vi "RW_main.vi"(0 "Rotating Wall Parameters":T1={"Start Frequency"=20000.0, "Stop Frequency"=20000.0, "Sweep Time"=0.0, "Amplitude"=1.5, "Phase (ch.1)"=0.001, "Phase (Ch.2)"=90.0} {"Sweep Time" format="%.4f"; "Phase (Ch.2)" min=-1800.0 max=1800.0 step=0.1 format="%.3f"; "Phase (ch.1)" min=-1800.0 max=1800.0 step=0.1 format="%.3f"; "Stop Frequency" format="%#.5p"; "Start Frequency" format="%#.5p"; "Amplitude" min=0.0 max=4.0 format="%.3f"}, 1 "On/Off":bool, 2 "VISAsession":refnum<visa-resource-name>="wavefactoryU10") -> ()   [LabVIEW 2018]
panel:
  out "x-y 5":u32=300
  out "x-y 4":u32=100
  out "x-y 3":u32=901
  out "x-y 2":u32=800
  out "x-y":u32=600
  out "millisecond timer value":u32=88672931
  out "error out":errorcluster caption="Error OUT"
  # "Turn-on\nTimes (ms)"
  # "Turn-off\nTimes (ms)"
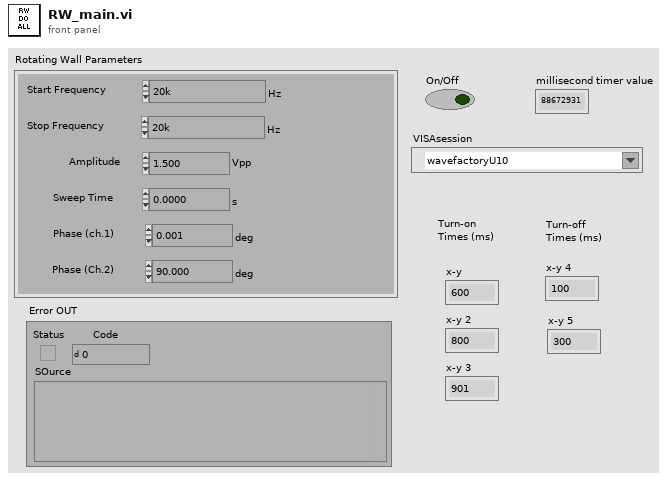
[diagram p1: front panel]
types:
  T1 = cluster{"Start Frequency":dbl, "Stop Frequency":dbl, "Sweep Time":dbl, "Amplitude":dbl, "Phase (ch.1)":dbl, "Phase (Ch.2)":dbl}
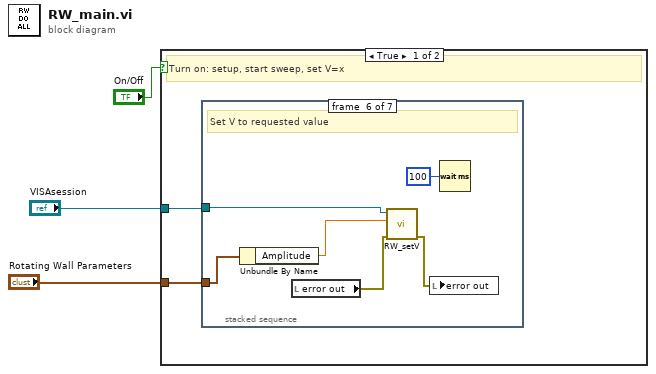
[diagram p0: block diagram]
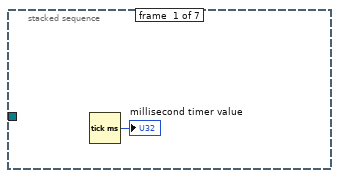
[diagram p2: hidden frame]
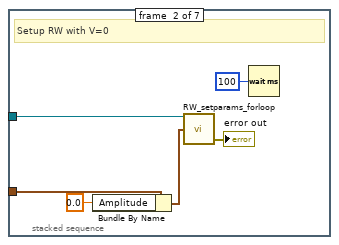
[diagram p3: hidden frame]
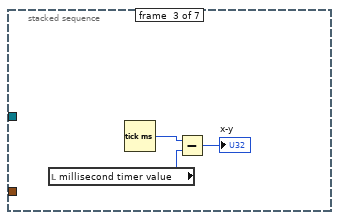
[diagram p4: hidden frame]
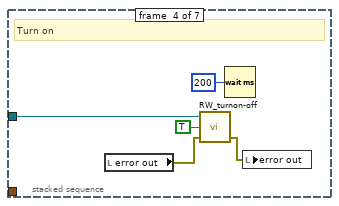
[diagram p5: hidden frame]
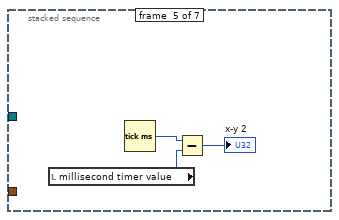
[diagram p6: hidden frame]
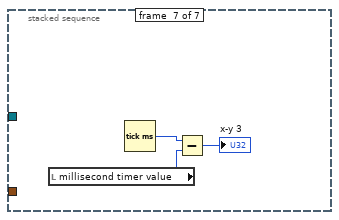
[diagram p7: hidden frame]
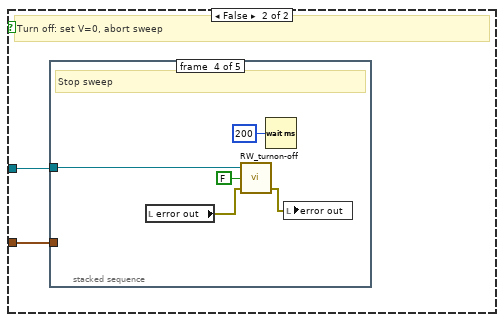
[diagram p8: hidden frame]
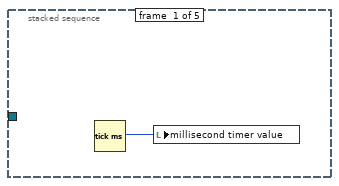
[diagram p9: hidden frame]
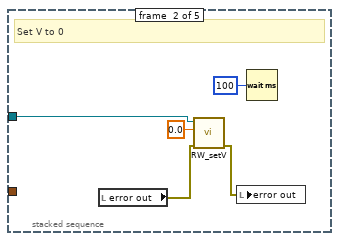
[diagram p10: hidden frame]
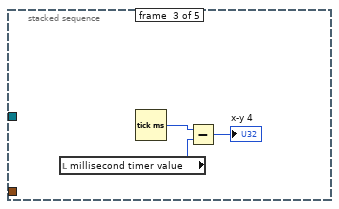
[diagram p11: hidden frame]
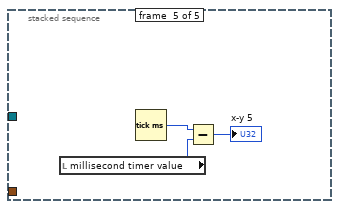
[diagram p12: hidden frame]
diagram:
  n1 = case shown="True" "On/Off" {
    tunnel: "Rotating Wall Parameters" -> [w5 w34]
    tunnel: "VISAsession" -> [w4 w33]
    frame True {
      # "Turn on: setup, start sweep, set V=x"
      n2 = stacked-sequence {
        tunnel: w4 -> [_ w12 _ w19 _ w29 _]
        tunnel: w5 -> [_ w8 _ _ _ w28 _]
        frame #0 {
          n3 = Tick Count (ms)() -> (millisecond timer value=→"millisecond timer value":u32)
        }
        frame #1 {
          # "Setup RW with V=0"
          n4 = Bundle By Name(cluster=w8, "Amplitude"=0.0) -> (w7:T1)
          n5 = call "RW_setparams_forloop.vi"("Rotating Wall Parameters"=w7, "VISAsession"=w12) -> ("error out"=→"error out":errorcluster)  [unwired: 2 in, 1 out]
          n6 = Wait (ms)(milliseconds to wait=u32 100) -> ()  [unwired: 1 out]
        }
        frame #2 {
          n7 = local read "millisecond timer value"() -> (w14:u32)
          n8 = Tick Count (ms)() -> (millisecond timer value=w15:u32)
          n9 = Subtract(x=w15, y=w14) -> (x-y=→"x-y":u32)
        }
        frame #3 {
          # "Turn on"
          n10 = local read "error out"() -> (w18:errorcluster)
          n11 = call "RW_turnon-off.vi"("error in (no error)"=w18, "On/Off"=TRUE, "VISAsession"=w19) -> ("error out"=w17:errorcluster)  [unwired: 1 in, 1 out]
          n12 = Wait (ms)(milliseconds to wait=u32 200) -> ()  [unwired: 1 out]
          n13 = local write "error out"(w17) -> ()
        }
        frame #4 {
          n14 = local read "millisecond timer value"() -> (w22:u32)
          n15 = Tick Count (ms)() -> (millisecond timer value=w23:u32)
          n16 = Subtract(x=w23, y=w22) -> (x-y=→"x-y 2":u32)
        }
        frame #5 {
          # "Set V to requested value"
          n17 = Unbundle By Name(w28) -> ("Amplitude"=w25:dbl)
          n18 = local read "error out"() -> (w27:errorcluster)
          n19 = call "RW_setV.vi"("error in (no error)"=w27, "voltage"=w25, "VISAsession"=w29) -> ("error out"=w26:errorcluster)  [unwired: 8 in]
          n20 = local write "error out"(w26) -> ()
          n21 = Wait (ms)(milliseconds to wait=u32 100) -> ()  [unwired: 1 out]
        }
        frame #6 {
          n22 = local read "millisecond timer value"() -> (w31:u32)
          n23 = Tick Count (ms)() -> (millisecond timer value=w32:u32)
          n24 = Subtract(x=w32, y=w31) -> (x-y=→"x-y 3":u32)
        }
      }
    }
    frame False {
      # "Turn off: set V=0, abort sweep"
      n25 = stacked-sequence {
        tunnel: w33 -> [_ w40 _ w47 _]
        tunnel: w34 -> [_ _ _ _ _]
        frame #0 {
          n26 = Tick Count (ms)() -> (millisecond timer value=w35:u32)
          n27 = local write "millisecond timer value"(w35) -> ()
        }
        frame #1 {
          # "Set V to 0"
          n28 = local read "error out"() -> (w39:errorcluster)
          n29 = call "RW_setV.vi"("error in (no error)"=w39, "voltage"=0.0, "VISAsession"=w40) -> ("error out"=w38:errorcluster)  [unwired: 8 in]
          n30 = local write "error out"(w38) -> ()
          n31 = Wait (ms)(milliseconds to wait=u32 100) -> ()  [unwired: 1 out]
        }
        frame #2 {
          n32 = local read "millisecond timer value"() -> (w42:u32)
          n33 = Tick Count (ms)() -> (millisecond timer value=w43:u32)
          n34 = Subtract(x=w43, y=w42) -> (x-y=→"x-y 4":u32)
        }
        frame #3 {
          # "Stop sweep"
          n35 = local read "error out"() -> (w46:errorcluster)
          n36 = call "RW_turnon-off.vi"("error in (no error)"=w46, "On/Off"=FALSE, "VISAsession"=w47) -> ("error out"=w45:errorcluster)  [unwired: 1 in, 1 out]
          n37 = Wait (ms)(milliseconds to wait=u32 200) -> ()  [unwired: 1 out]
          n38 = local write "error out"(w45) -> ()
        }
        frame #4 {
          n39 = local read "millisecond timer value"() -> (w50:u32)
          n40 = Tick Count (ms)() -> (millisecond timer value=w51:u32)
          n41 = Subtract(x=w51, y=w50) -> (x-y=→"x-y 5":u32)
        }
      }
    }
  }
